vi "DAQmx Timing (Use Waveform).vi"(0 "task/channels in":refnum<k21>, 1 "sample mode":i32(ring)=10178 items=["Finite Samples"=10178, "Continuous Samples"=10123, "Hardware Timed Single Point"=12522], 5 "waveform":waveform(dbl)={"t0"=timestamp(0 s since 1904-01-01), "dt"=0.0, "Y"=[]}, 11 "error in":errorcluster) -> (4 "task out":refnum<k21>, 15 "error out":errorcluster)   [LabVIEW 2013]
doc: "Uses the <B>dt</B> component of the <B>waveform</B> input to determine the Sample Clock rate. <B>dt</B> is the time in seconds between samples. If <B>sample mode</B> is <B>Finite Samples</B>, NI-DAQmx generates the number of samples in the waveform. This VI does not actually generate any samples. You must wire the same waveform to the DAQmx Write VI to generate the samples."
uses:
  nilvaiu.dll
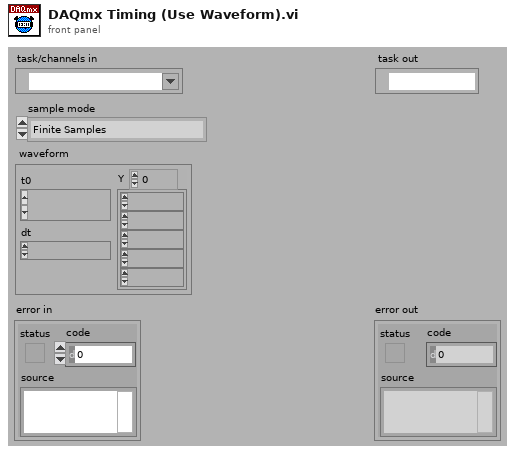
[diagram p1: front panel]
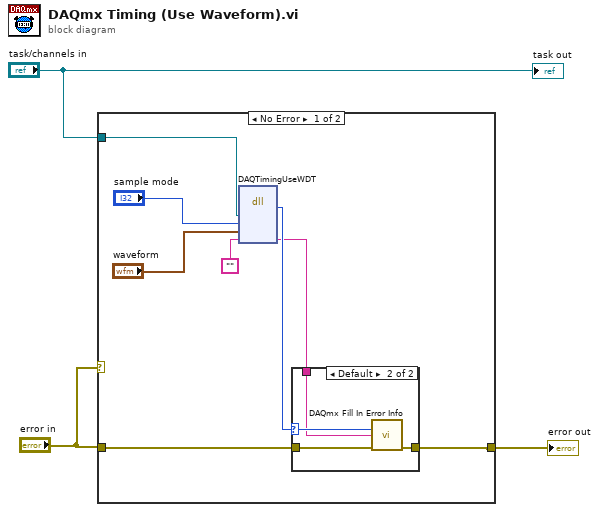
[diagram p0: block diagram]
diagram:
  n1 = case shown="No Error" "error in" {
    tunnel: [w8 w17] -> w1
    tunnel: "error in" -> [w10 w17]
    tunnel: "task/channels in" -> [w11 _]
    frame No Error {
      n2 = dll-call lib="nilvaiu.*" fn="DAQTimingUseWDT"("taskID"=w11, "sampleMode"="sample mode", "waveform"="waveform", "extendedErrorInfo"="") -> (w9:i32, "extendedErrorInfo"=w4:string)  [unwired: 5 in, 3 out]
      n3 = case shown="Default" w9 {
        selector: w9 -> [_ w14]
        tunnel: w10 -> [w12 w16]
        tunnel: [w12 w15] -> w8
        tunnel: w4 -> [_ w13]
        frame 0 {
        }
        frame Default {
          n4 = call "DAQmx Fill In Error Info.vi"("status code"=w14, "extended error info"=w13, "error in"=w16) -> ("error out"=w15:errorcluster)  [unwired: 1 in, 11 out]
        }
      }
    }
    frame Error {
    }
  }
  "error out" <- w1
  "task out" <- "task/channels in"
